vi "GetConfigFromFile.vi"(8 "error in (no error)":errorcluster, 11 "Config File":path) -> (0 "error out":errorcluster, 3 "Config":T1={"LogName"="", "Level"=enum."Info", "LogFolder"=path "", "MaxFileSize"=0, "FileExtension"="", "TimeSytle"="", "LogStyle"=""})   [LabVIEW 2016, in "Log4Lv.lvlib"]
doc: "Use this template to build a VI to use as a subVI."
uses:
  Log4Lv.lvlib
  <vilib>/Utility/config.llb/Read Key (String).vi
  <vilib>/Utility/config.llb/Read Key (Path).vi
  <vilib>/Utility/config.llb/Read Key (I32).vi
  <vilib>/Utility/config.llb/NI_LVConfig.lvlib
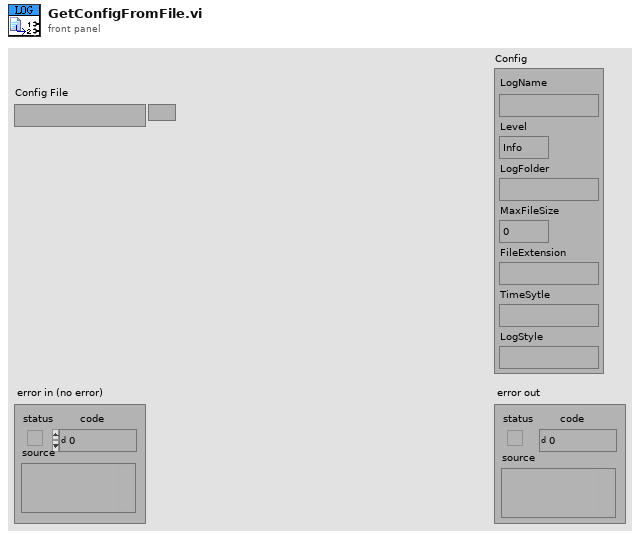
[diagram p1: front panel]
types:
  T1 = cluster{"LogName":string, "Level":enum16{"Disable", "Error", "Warn", "Info", "Debug"}, "LogFolder":path, "MaxFileSize":i32, "FileExtension":string, "TimeSytle":string, "LogStyle":string}
  T2 = enum16{"Disable", "Error", "Warn", "Info", "Debug"}
  T3 = typedef "NI_LVConfig.lvlib/Config Data RefNum.ctl" = refnum<k1>
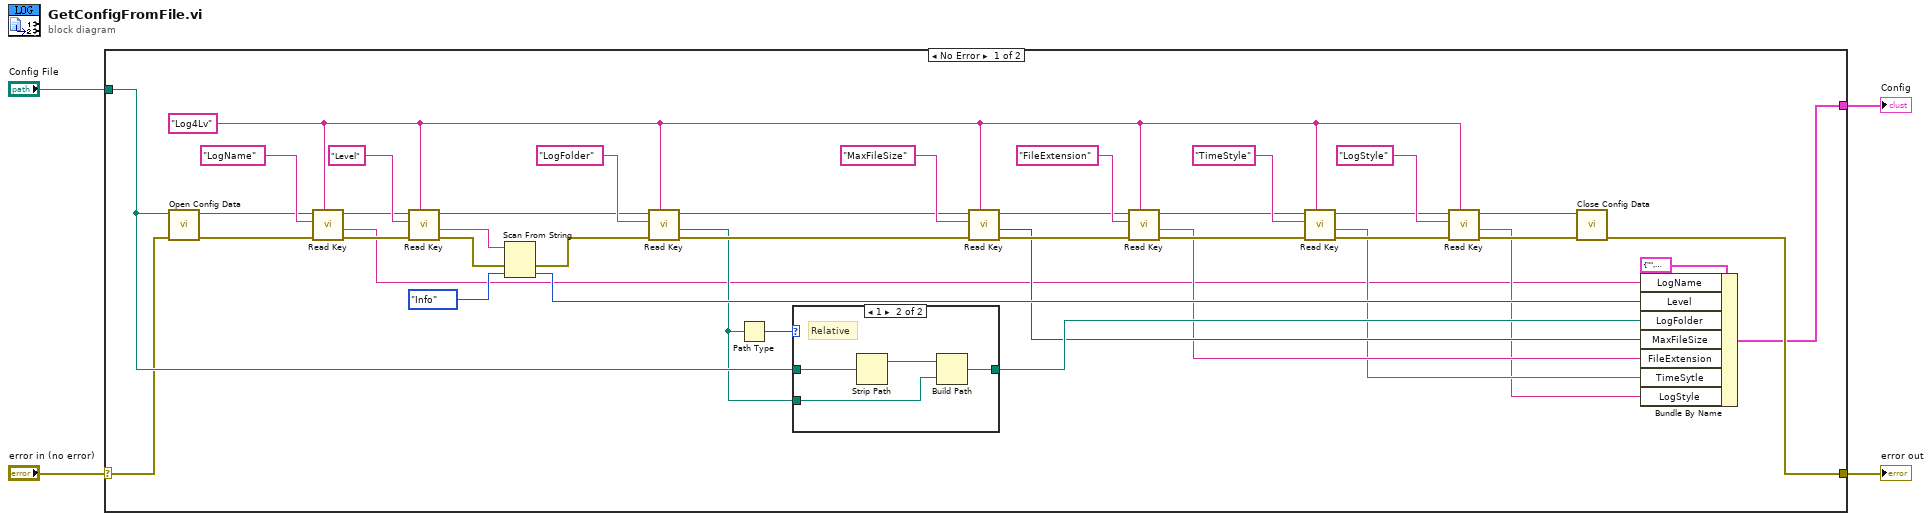
[diagram p0: block diagram]
diagram:
  n1 = case shown="No Error" "error in (no error)" {
    selector: "error in (no error)" -> [w15 w51]
    tunnel: [w16 w51] -> w2
    tunnel: "Config File" -> [w23 _]
    tunnel: [w13 _] -> w1
    frame No Error {
      w6 = "Log4Lv" ("section")
      n2 = call <vilib>:"Open Config Data.vi"("error in (no error)"=w15, "configuration file path"=w23) -> ("error out"=w8:errorcluster, "refnum"=w10:T3)  [unwired: 7 in, 1 out]
      n3 = call-poly <vilib>:"Read Key.vi"("section"=w6, "error in (no error)"=w8, "key"="LogName", "refnum"=w10) -> ("error out"=w7:errorcluster, "value"=w5:string, "refnum out"=w9:T3)  [unwired: 4 in, 1 out]
      n4 = call-poly <vilib>:"Read Key.vi"("section"=w6, "error in (no error)"=w7, "key"="Level", "refnum"=w9) -> ("error out"=w41:errorcluster, "value"=w14:string, "refnum out"=w40:T3)  [unwired: 4 in, 1 out]
      n5 = Scan From String "Scan From String"(input string=w14, error in=w41, default 1=T2."Info" ("Level")) -> (error out=w39:errorcluster, output 1=w25:T2)  [unwired: 2 in, 2 out]
      n6 = call-poly <vilib>:"Read Key.vi"("section"=w6, "error in (no error)"=w39, "key"="LogFolder", "refnum"=w40) -> ("error out"=w37:errorcluster, "value"=w22:path, "refnum out"=w38:T3)  [unwired: 4 in, 1 out]
      n7 = Path Type(1:w22) -> (0:w24:i16)
      n8 = case shown="1" w24 {
        tunnel: w23 -> [_ w50]
        tunnel: w22 -> [w46 w48]
        tunnel: [w46 w47] -> w21
        frame 0, Default {
          # "Absolute"
        }
        frame 1 {
          # "Relative"
          n9 = Strip Path(path=w50) -> (stripped path=w49:path)  [unwired: 1 out]
          n10 = Build Path(base path=w49, name or relative path=w48) -> (appended path=w47:path)
        }
      }
      n11 = call-poly <vilib>:"Read Key.vi"("section"=w6, "error in (no error)"=w37, "key"="MaxFileSize", "refnum"=w38) -> ("error out"=w34:errorcluster, "value"=w20:i32, "refnum out"=w33:T3)  [unwired: 4 in, 1 out]
      n12 = call-poly <vilib>:"Read Key.vi"("section"=w6, "error in (no error)"=w34, "key"="FileExtension", "refnum"=w33) -> ("error out"=w31:errorcluster, "value"=w19:string, "refnum out"=w32:T3)  [unwired: 4 in, 1 out]
      n13 = call-poly <vilib>:"Read Key.vi"("section"=w6, "error in (no error)"=w31, "key"="TimeStyle", "refnum"=w32) -> ("error out"=w26:errorcluster, "value"=w18:string, "refnum out"=w27:T3)  [unwired: 4 in, 1 out]
      n14 = call-poly <vilib>:"Read Key.vi"("section"=w6, "error in (no error)"=w26, "key"="LogStyle", "refnum"=w27) -> ("error out"=w30:errorcluster, "value"=w17:string, "refnum out"=w29:T3)  [unwired: 4 in, 1 out]
      n15 = call <vilib>:"Close Config Data.vi"("error in (no error)"=w30, "refnum"=w29) -> ("error out"=w16:errorcluster)  [unwired: 8 in, 1 out]
      n16 = Bundle By Name(cluster=T1 {"LogName"="", "Level"=enum."Info", "LogFolder"=path "", "MaxFileSize"=0, "FileExtension"="", "TimeSytle"="", "LogStyle"=""} ("Config"), "LogName"=w5, "Level"=w25, "LogFolder"=w21, "MaxFileSize"=w20, "FileExtension"=w19, "TimeSytle"=w18, "LogStyle"=w17) -> (w13:T1)
    }
    frame Error {
    }
  }
  "error out" <- w2
  "Config" <- w1
